vi "Instr Config.vi"(8 "error constant":errorcluster, 11 "Configuration":string) -> (0 "error out":errorcluster)   [LabVIEW 2024, in "Setting_Screen.lvlib"]
uses:
  Setting_Screen.lvlib
  support/Combined_Instrs.ctl
  support/Comb_instr_names.ctl
  support/Common_Equips.ctl
  support/Instr_Cluster.ctl
  support/Instr_enum.ctl
  Launcher/Launcher_DTU.lvlib
panel:
  in  "Exit":bool
  in  "Save":bool
  in  "Common Equip Config":cluster{"Common_Equip ":T1, "COMM/IP ":string}[](array[cluster])
  in  "Combined Equip Config":T4(array[cluster])
  in  "CombinedEquip Row To Change :":u8
  # "INSTRUMENT CONFIGURATIONS"
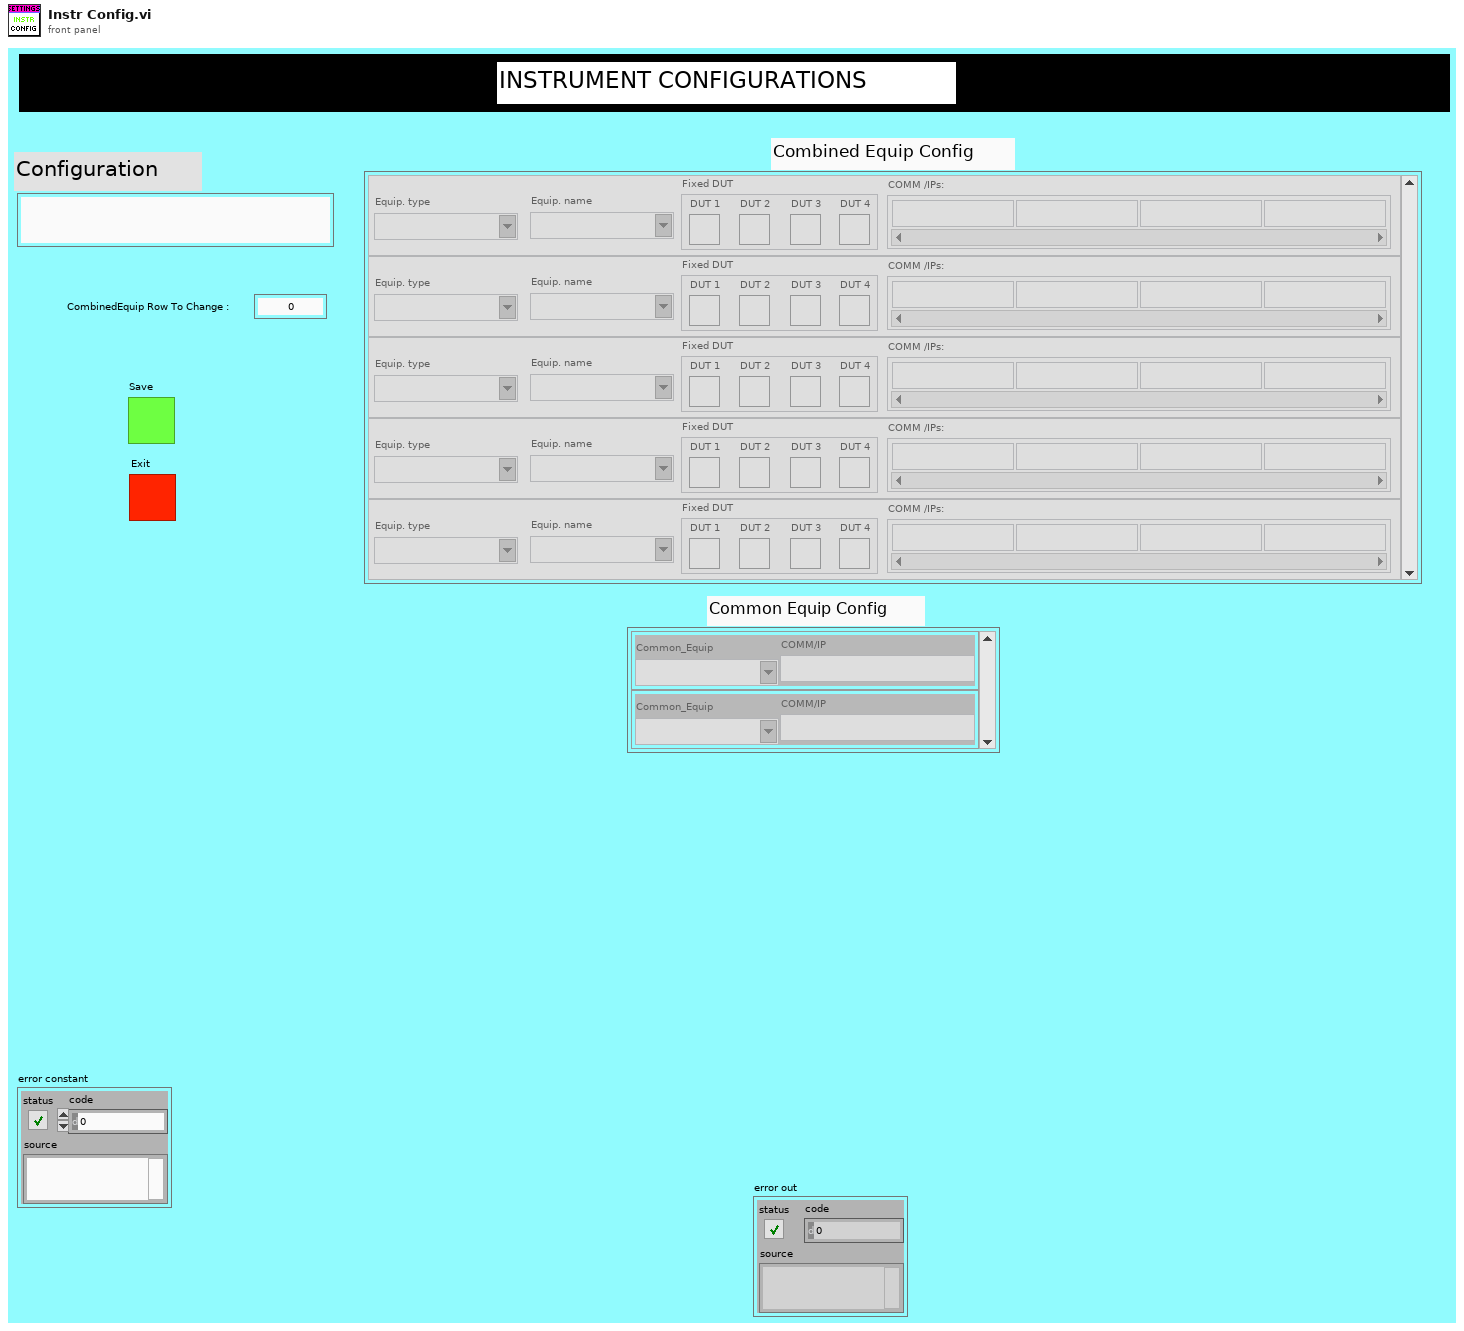
[diagram p1: front panel]
types:
  T1 = typedef "Setting_Screen.lvlib/Common_Equips.ctl" = string
  T2 = typedef "Setting_Screen.lvlib/Combined_Instrs.ctl" = string
  T3 = typedef "Setting_Screen.lvlib/Comb_instr_names.ctl" = string
  T4 = cluster{"Equip. type ":T2, "Equip. name":T3, "Fixed DUT":cluster{"DUT 1":bool, "DUT 2":bool, "DUT 3":bool, "DUT 4":bool}, "COMM /IPs:":string[]}[]
  T5 = typedef "Setting_Screen.lvlib/Instr_enum.ctl" = enum16{"Init", "Poll", "Read Config", "New Config", "Save", "Update Display", "Exit"}
  T6 = typedef "Setting_Screen.lvlib/Instr_Cluster.ctl" = cluster{"Common _eqip pth":path, "Combined _eqip pth":path, "CombinedEquip Row To Change : ":u8, "Combined Equip Config":cluster{"Equip. type ":T2, "Equip. name":T3, "Fixed DUT":cluster{"DUT 1":bool, "DUT 2":bool, "DUT 3":bool, "DUT 4":bool}, "COMM /IPs:":string[]}[], "Common Equip Config":cluster{"Common_Equip ":T1, "COMM/IP ":string}[]}
  T7 = enum16{"Read", "Write", "All_sections", "All_values", "Remove key&section"}
  T8 = cluster{"Equip. type ":T2, "Equip. name":T3, "Fixed DUT":cluster{"DUT 1":bool, "DUT 2":bool, "DUT 3":bool, "DUT 4":bool}, "COMM /IPs:":string[]}
  T9 = cluster{"[0]":bool, "[1]":bool, "[2]":bool, "[3]":bool}
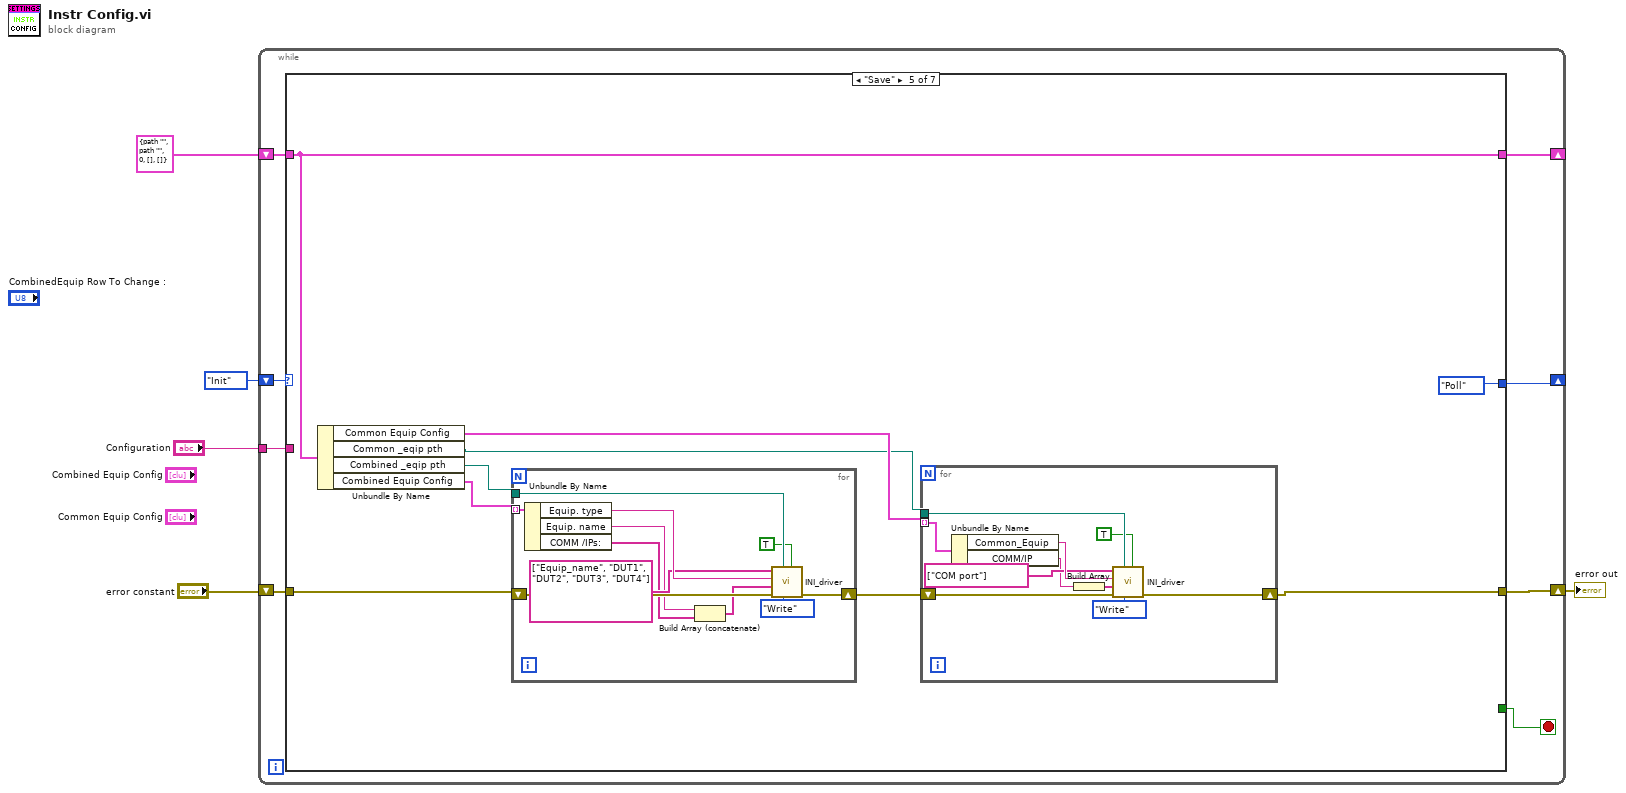
[diagram p0: block diagram]
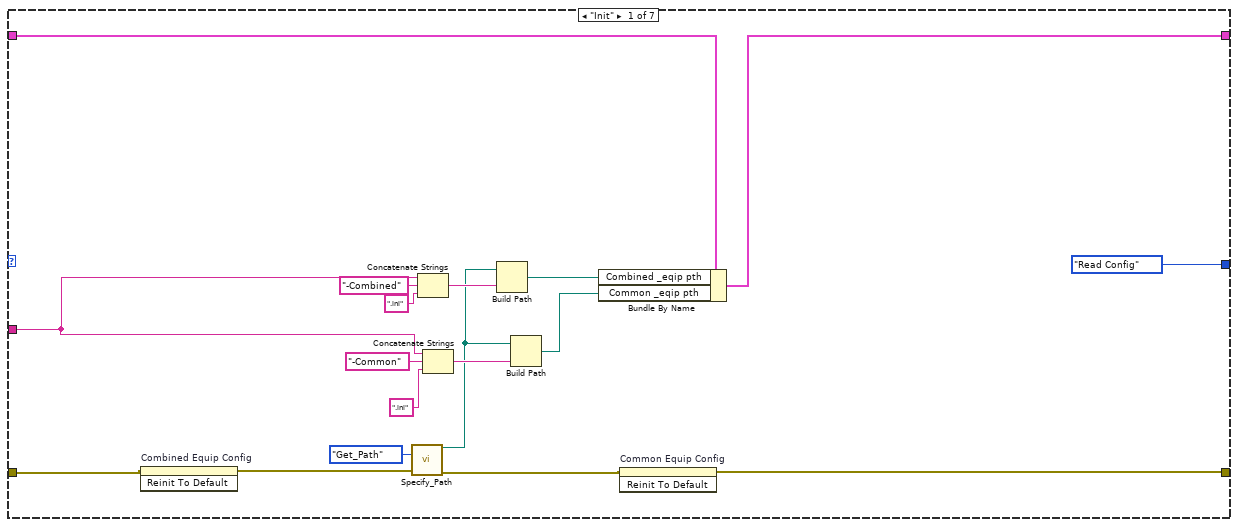
[diagram p2: hidden frame]
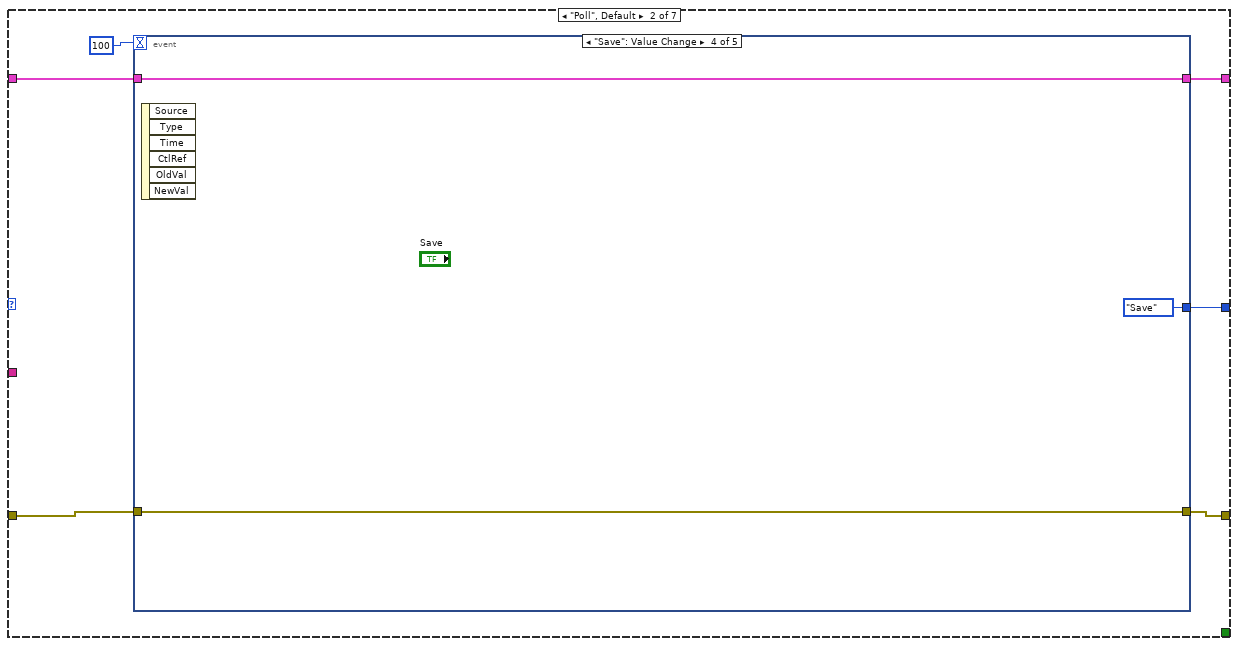
[diagram p3: hidden frame]
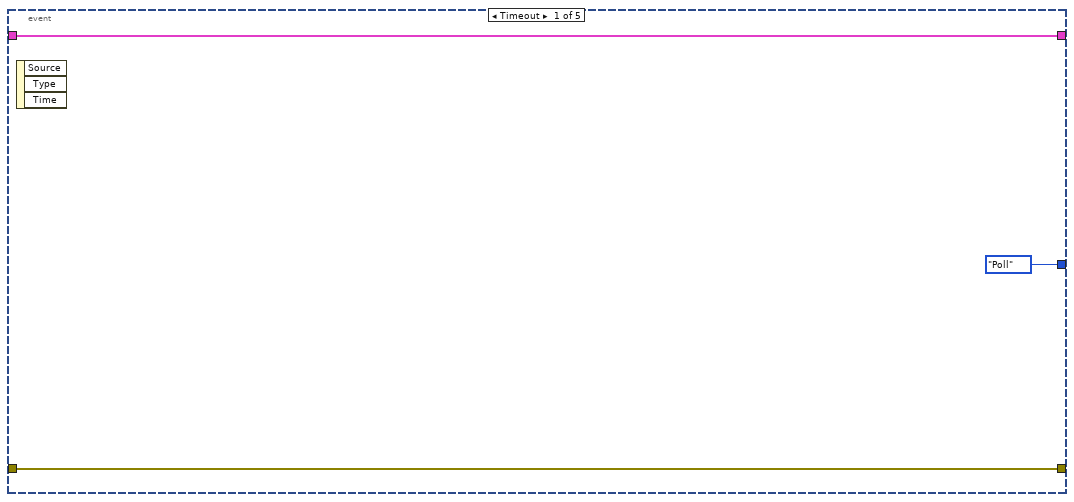
[diagram p4: hidden frame]
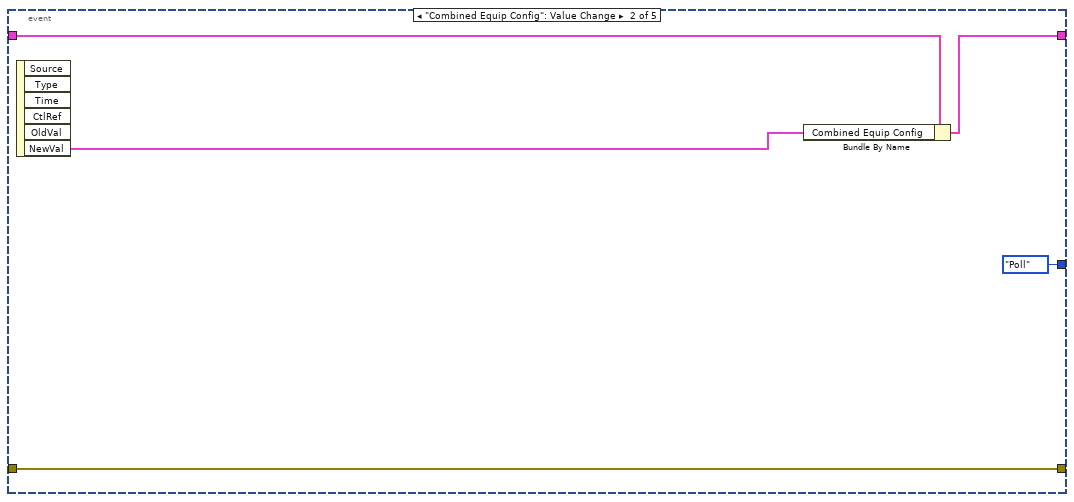
[diagram p5: hidden frame]
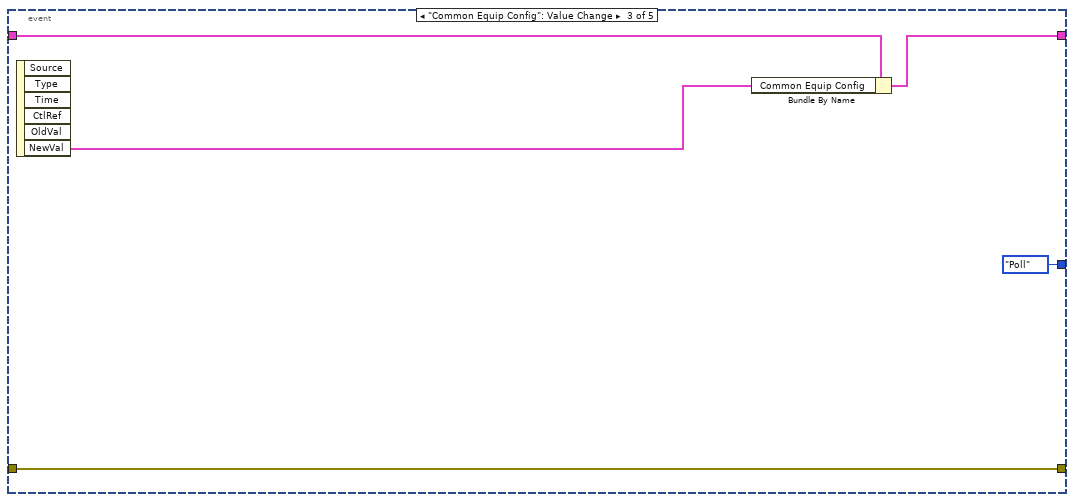
[diagram p6: hidden frame]
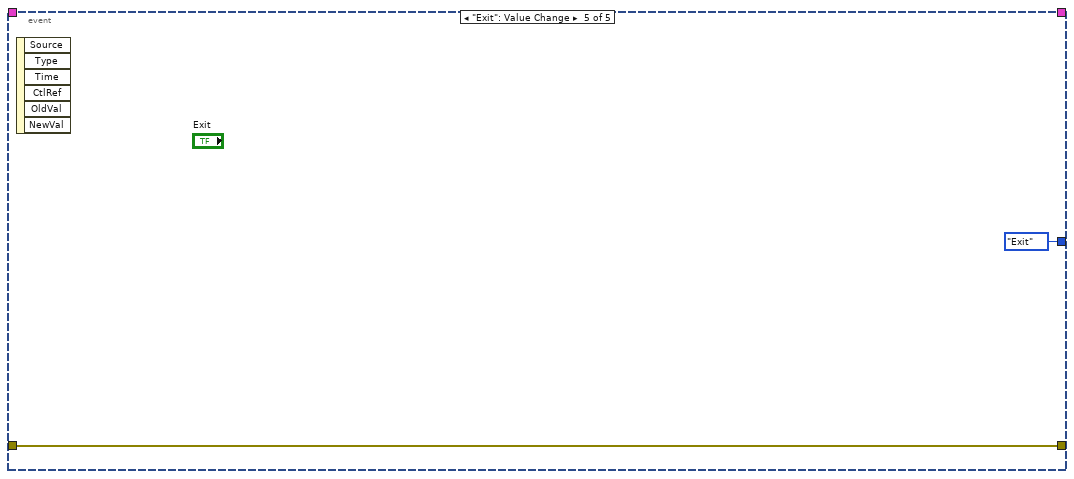
[diagram p7: hidden frame]
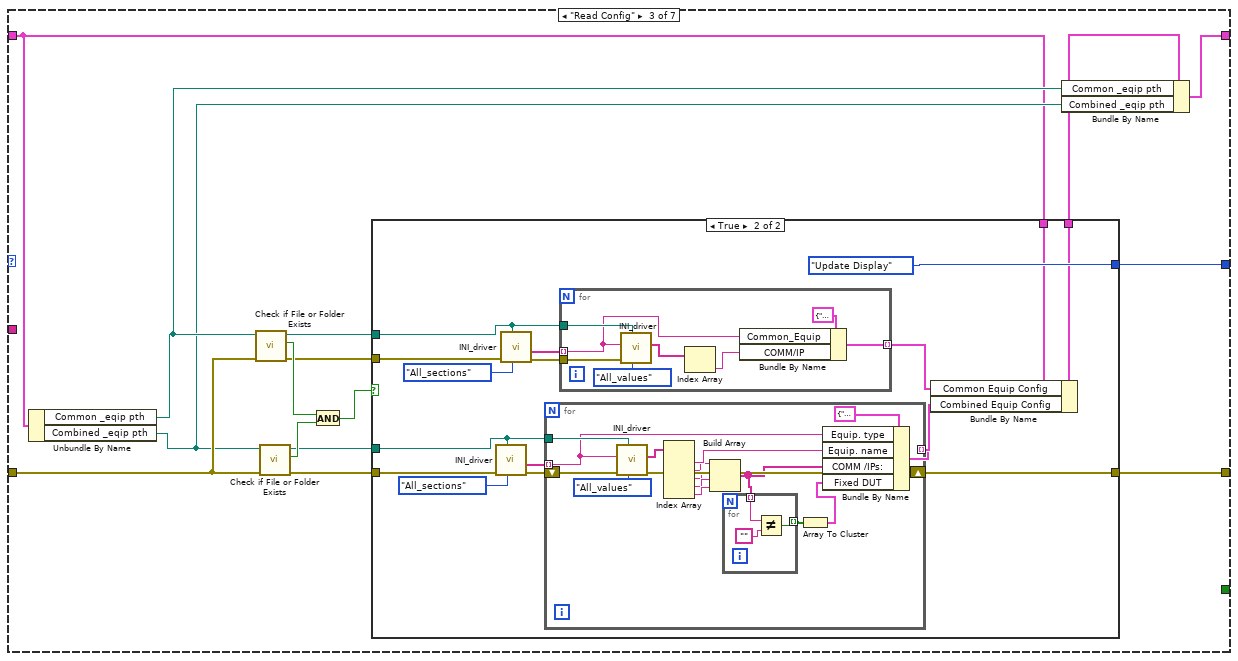
[diagram p8: hidden frame]
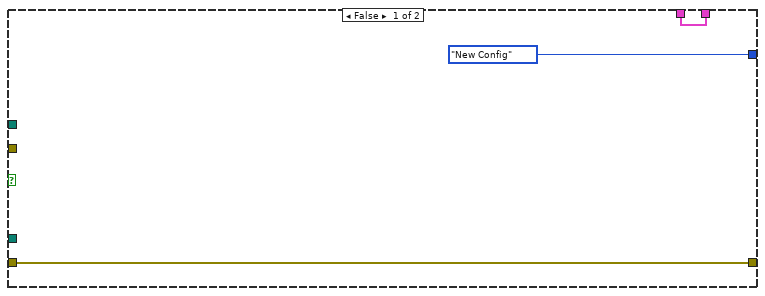
[diagram p9: hidden frame]
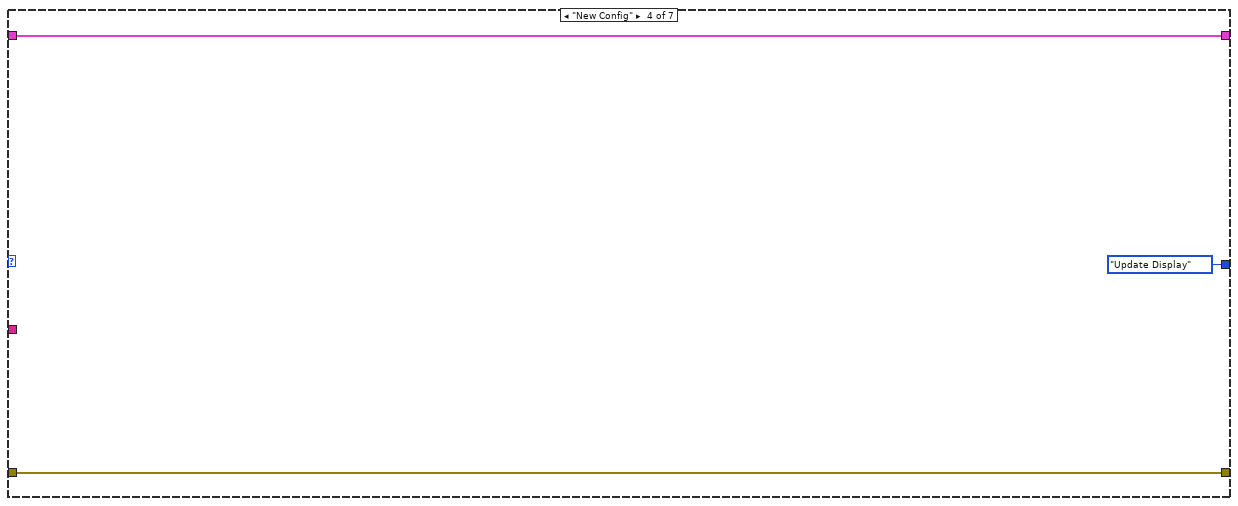
[diagram p10: hidden frame]
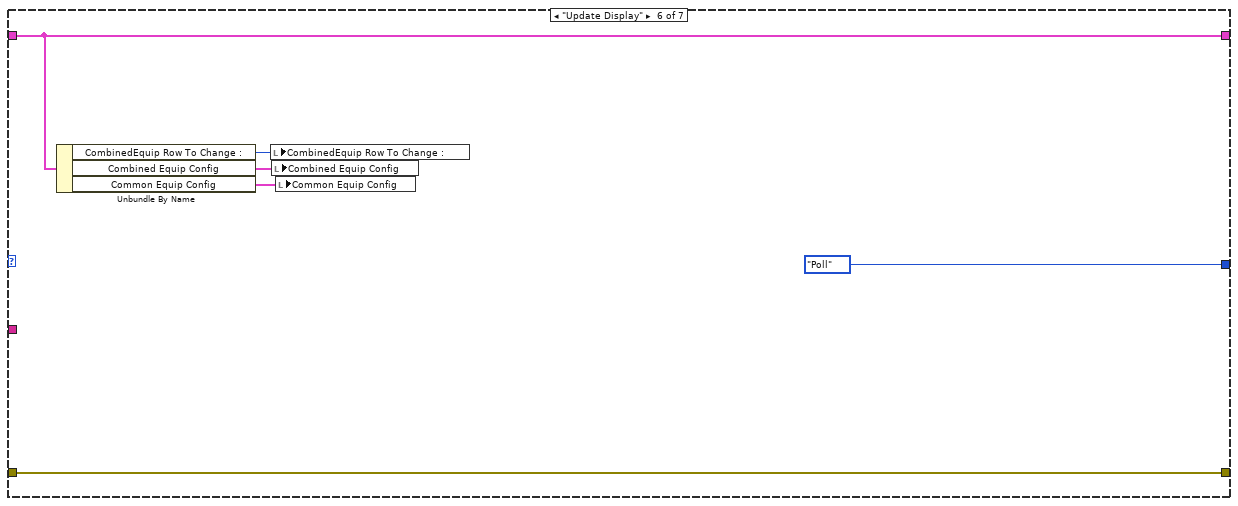
[diagram p11: hidden frame]
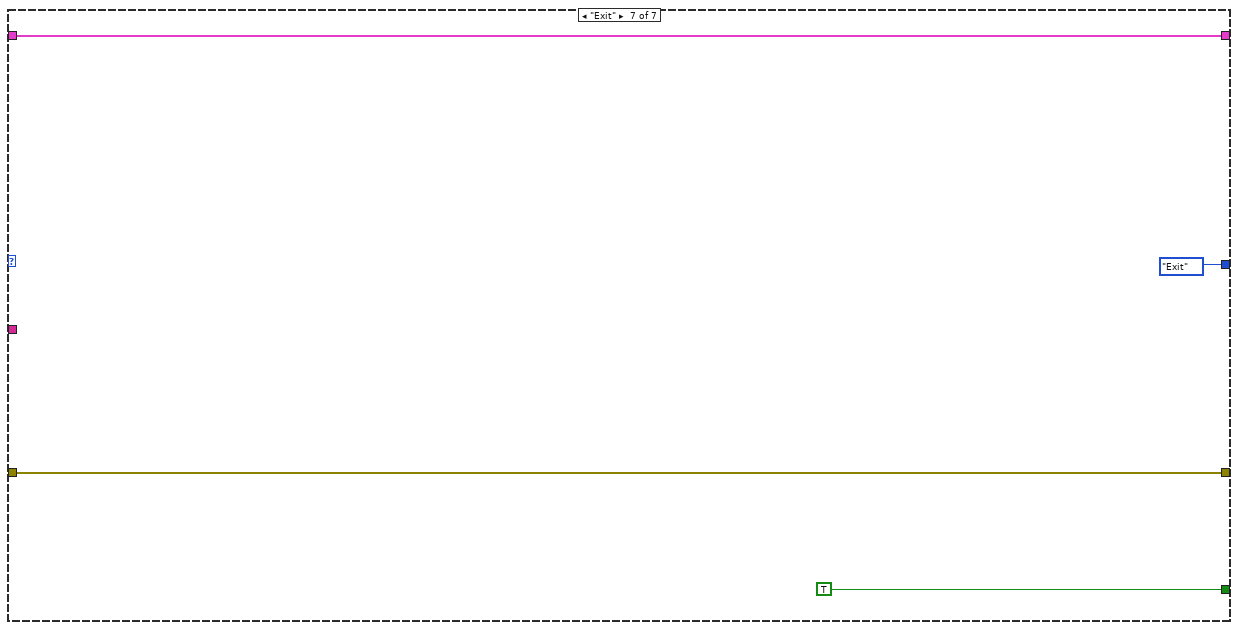
[diagram p12: hidden frame]
diagram:
  n1 = while {
    shift-right: [w9] -> _
    shift-left: T6 {"Common _eqip pth"=path "", "Combined _eqip pth"=path "", "CombinedEquip Row To Change : "=0, "Combined Equip Config"=[], "Common Equip Config"=[]} -> [w13]
    shift-right: [w10] -> w1
    shift-left: "error constant" -> [w11]
    shift-right: [w8] -> _
    shift-left: Instr_enum."Init" -> [w12]
    tunnel: "Configuration" -> [w7]
    stop <- w6 stop-if-true
    n2 = case shown="\"Save\"" w12 {
      tunnel: w13 -> [w30 w36 w59 w117 w120 w153 w156]
      tunnel: w11 -> [w18 w33 w70 w118 w127 w154 w158]
      tunnel: [w15 w34 w60 w118 w121 w154 w158] -> w10
      tunnel: [w28 w35 w63 w117 w120 w153 w156] -> w9
      tunnel: [Instr_enum."Read Config" w32 w66 Instr_enum."Update Display" Instr_enum."Poll" Instr_enum."Poll" Instr_enum."Exit"] -> w8
      tunnel: w7 -> [w14 _ _ _ _ _ _]
      tunnel: [_ _ _ _ _ _ TRUE] -> w6
      frame "Init" {
        n3 = invoke on="Combined Equip Config" class="Arr (strict)" method="Reinit To Default"(error in=w18) -> (error out=w17:errorcluster)  [unwired: 2 in, 2 out]
        n4 = call "Specify_Path.vi"("Path_Enum"=enum16{"Find_Path", "Get_Path"}."Get_Path", "error in (no error)"=w17) -> ("Configurations"=w21:path, "error out"=w16:errorcluster)  [unwired: 6 in, 6 out]
        n5 = Concatenate Strings(w14, "-Combined" ("string"), ".ini" ("string")) -> (w22:string)
        n6 = Concatenate Strings(w14, "-Common" ("string"), ".ini" ("string")) -> (w23:string)
        n7 = Build Path(base path=w21, name or relative path=w22) -> (appended path=w20:path)
        n8 = Build Path(base path=w21, name or relative path=w23) -> (appended path=w19:path)
        n9 = Bundle By Name(cluster=w30, "Combined _eqip pth"=w20, "Common _eqip pth"=w19) -> (w28:T6)
        n10 = invoke on="Common Equip Config" class="Arr (strict)" method="Reinit To Default"(error in=w16) -> (error out=w15:errorcluster)  [unwired: 2 in, 2 out]
      }
      frame "Poll", Default {
        n11 = event shown="[3] \"Save\": Value Change" {
          selector: _ -> [_ _ _ _ _]
          dyn-events: _ -> [_ _ _ _ _]
          timeout: 100 -> [_ _ _ _ _]
          tunnel: w36 -> [w40 w45 w50 w53 _]
          tunnel: [w40 w44 w49 w53 _] -> w35
          tunnel: [w39 w42 w47 w51 w55] -> w34
          tunnel: w33 -> [w39 w42 w47 w51 w55]
          tunnel: [Instr_enum."Poll" Instr_enum."Poll" Instr_enum."Poll" Instr_enum."Save" Instr_enum."Exit"] -> w32
          event Timeout {
            n12 = event-data() -> ()  [unwired: 1 in, 3 out]
          }
          event "Combined Equip Config": Value Change {
            n13 = event-data() -> ("NewVal"=w43:T4)  [unwired: 1 in, 5 out]
            n14 = Bundle By Name(cluster=w45, "Combined Equip Config"=w43) -> (w44:T6)
          }
          event "Common Equip Config": Value Change {
            n15 = event-data() -> ("NewVal"=w46:cluster{"Common_Equip ":T1, "COMM/IP ":string}[])  [unwired: 1 in, 5 out]
            n16 = Bundle By Name(cluster=w50, "Common Equip Config"=w46) -> (w49:T6)
          }
          event "Save": Value Change {
            n17 = event-data() -> ()  [unwired: 1 in, 6 out]
          }
          event "Exit": Value Change {
            n18 = event-data() -> ()  [unwired: 1 in, 6 out]
          }
        }
      }
      frame "Read Config" {
        n19 = Unbundle By Name(w59) -> ("Common _eqip pth"=w62:path, "Combined _eqip pth"=w61:path)
        n20 = call <vilib>:"Check if File or Folder Exists.vi"("error in (no error)"=w70, "path"=w62) -> ("error out"=w65:errorcluster, "file or folder exists?"=w69:bool, "dup path"=w57:path)  [unwired: 7 in]
        n21 = call <vilib>:"Check if File or Folder Exists.vi"("error in (no error)"=w70, "path"=w61) -> ("error out"=w64:errorcluster, "file or folder exists?"=w68:bool, "dup path"=w56:path)  [unwired: 7 in]
        n22 = And(x=w69, y=w68) -> (x .and. y?=w67:bool)
        n23 = case shown="True" w67 {
          tunnel: [Instr_enum."New Config" Instr_enum."Update Display"] -> w66
          tunnel: w65 -> [_ w86]
          tunnel: w64 -> [w72 w85]
          tunnel: [w72 w79] -> w60
          tunnel: w59 -> [w71 w88]
          tunnel: [w71 w87] -> w58
          tunnel: w57 -> [_ w76]
          tunnel: w56 -> [_ w78]
          frame False {
          }
          frame True {
            n24 = call "INI_driver.vi"("Enum"=T7."All_sections", "instrument file path"=w78, "error in (no error)"=w85) -> ("error out"=w80:errorcluster, "section names"=w82:string[])  [unwired: 5 in, 2 out]
            n25 = call "INI_driver.vi"("Enum"=T7."All_sections", "instrument file path"=w76, "error in (no error)"=w86) -> ("error out"=w77:errorcluster, "section names"=w83:string[])  [unwired: 5 in, 2 out]
            n26 = for {
              tunnel: w82 -> [w100] mode=indexing
              shift-right: [w104] -> w79
              shift-left: w80 -> [w105]
              tunnel: w78 -> [w103]
              tunnel: [w93] -> w75 mode=indexing
              n27 = call "INI_driver.vi"("Enum"=T7."All_values", "instrument file path"=w103, "error in (no error)"=w105, "Section"=w100) -> ("error out"=w104:errorcluster, "Values out"=w99:string[])  [unwired: 4 in, 2 out]
              n28 = Index Array(array=w99) -> (element #1=w98:string, element #2=w94:string, element #3=w95:string, element #4=w96:string, element #5=w97:string)  [unwired: 5 in]
              n29 = Build Array(w94, w95, w96, w97) -> (w92:string[])
              n30 = for {
                tunnel: w92 -> [w107] mode=indexing
                tunnel: [w106] -> w91 mode=indexing
                n31 = Not Equal?(x=w107, y="") -> (x != y?=w106:bool)
              }
              n32 = Array To Cluster(array=w91) -> (cluster=w90:T9)
              n33 = Bundle By Name(cluster=T8 {"Equip. type "="", "Equip. name"="", "Fixed DUT"={"DUT 1"=FALSE, "DUT 2"=FALSE, "DUT 3"=FALSE, "DUT 4"=FALSE}, "COMM /IPs:"=[]} ("Combined Equip Config"), "Equip. type"=w100, "Equip. name"=w98, "COMM /IPs:"=w92, "Fixed DUT"=w90) -> (w93:T8)
            }
            n34 = for {
              tunnel: w83 -> [w113] mode=indexing
              tunnel: w77 -> [w116]
              tunnel: w76 -> [w115]
              tunnel: [w112] -> w74 mode=indexing
              n35 = call "INI_driver.vi"("Enum"=T7."All_values", "instrument file path"=w115, "error in (no error)"=w116, "Section"=w113) -> ("Values out"=w110:string[])  [unwired: 4 in, 3 out]
              n36 = Index Array(array=w110) -> (element=w109:string)  [unwired: 1 in]
              n37 = Bundle By Name(cluster=cluster{"Common_Equip ":T1, "COMM/IP ":string} {"Common_Equip "="", "COMM/IP "=""} ("Cluster"), "Common_Equip"=w113, "COMM/IP"=w109) -> (w112:cluster{"Common_Equip ":T1, "COMM/IP ":string})
            }
            n38 = Bundle By Name(cluster=w88, "Common Equip Config"=w74, "Combined Equip Config"=w75) -> (w87:T6)
          }
        }
        n39 = Bundle By Name(cluster=w58, "Common _eqip pth"=w62, "Combined _eqip pth"=w61) -> (w63:T6)
      }
      frame "New Config" {
      }
      frame "Save" {
        n40 = Unbundle By Name(w120) -> ("Common Equip Config"=w124:cluster{"Common_Equip ":T1, "COMM/IP ":string}[], "Common _eqip pth"=w123:path, "Combined _eqip pth"=w126:path, "Combined Equip Config"=w125:T4)
        n41 = for {
          tunnel: w126 -> [w147]
          tunnel: w125 -> [w145] mode=indexing
          shift-right: [w139] -> w122
          shift-left: w127 -> [w149]
          n42 = Unbundle By Name(w145) -> ("Equip. type"=w144:T2, "Equip. name"=w141:T3, "COMM /IPs:"=w142:string[])
          n43 = Build Array (concatenate)(w141, w142) -> (w140:T3[])
          n44 = call "INI_driver.vi"("create file if necessary (T)"=TRUE, "Enum"=T7."Write", "instrument file path"=w147, "error in (no error)"=w149, "Value_in"=w140, "Section"=w144, "Key_name"=string[] ["Equip_name", "DUT1", "DUT2", "DUT3", "DUT4"]) -> ("error out"=w139:errorcluster)  [unwired: 1 in, 3 out]
        }
        n45 = for {
          tunnel: w124 -> [w136] mode=indexing
          tunnel: w123 -> [w138]
          shift-right: [w131] -> w121
          shift-left: w122 -> [w133]
          n46 = Unbundle By Name(w136) -> ("Common_Equip"=w135:T1, "COMM/IP"=w130:string)
          n47 = Build Array(w130) -> (w129:string[])
          n48 = call "INI_driver.vi"("create file if necessary (T)"=TRUE, "Enum"=T7."Write", "instrument file path"=w138, "error in (no error)"=w133, "Value_in"=w129, "Section"=w135, "Key_name"=string[] ["COM port"]) -> ("error out"=w131:errorcluster)  [unwired: 1 in, 3 out]
        }
      }
      frame "Update Display" {
        n49 = Unbundle By Name(w153) -> ("CombinedEquip Row To Change :"=w151:u8, "Combined Equip Config"=w150:T4, "Common Equip Config"=w152:cluster{"Common_Equip ":T1, "COMM/IP ":string}[])
        n50 = local write "CombinedEquip Row To Change :"(w151) -> ()
        n51 = local write "Combined Equip Config"(w150) -> ()
        n52 = local write "Common Equip Config"(w152) -> ()
      }
      frame "Exit" {
      }
    }
  }
  "error out" <- w1
